vi "New Event Transport.vi"(10 "Event Priority (normal)":T1) -> (0 "error out":errorcluster, 2 "Tranport Event":refnum<user-event>, 3 "EventTransport Out":refnum<class "EventTransport.lvclass">)   [LabVIEW 2015, in "Mediator.lvlib" / "EventTransport.lvclass"]
doc: "<License>\nCopyright © 2017 Composed Systems, LLC | All rights reserved\nwww.composed.io\n\nAuthor: Ethan Stern <ethan.stern@composed.io>\n\nThis software is provided \"AS IS\" WITHOUT WARRANTIES, either express or implied, AND IS FOR EDUCATIONAL PURPOSES ONLY.\n</License>"
uses:
  EventTransport.lvclass
  <vilib>/event_ctls.llb/usereventprio.ctl
  EventTransport.lvclass/EventTransport.ctl
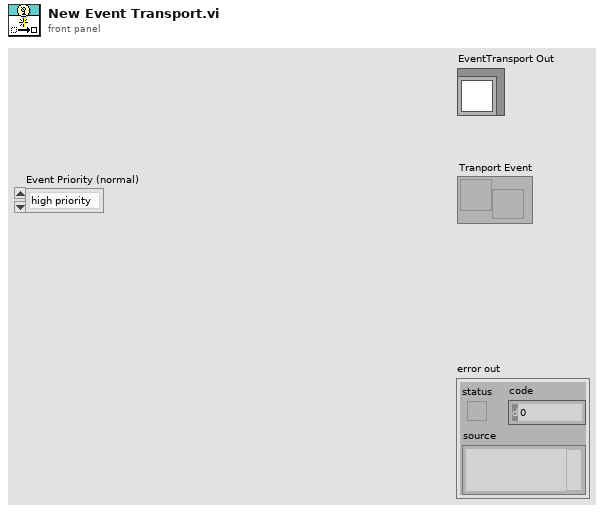
[diagram p1: front panel]
types:
  T1 = typedef "usereventprio.ctl" = enum32{"high priority", "normal priority"}
  T2 = cluster{"Data":variant, "Publication Time":timestamp}
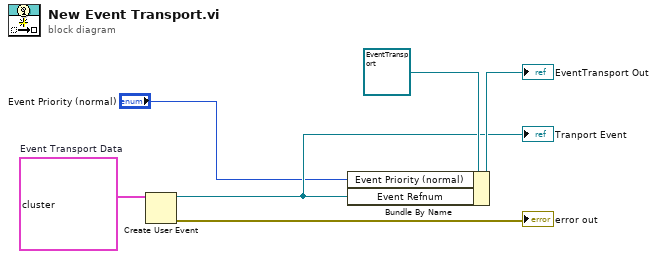
[diagram p0: block diagram]
diagram:
  w3 = T2 {"Data"=variant, "Publication Time"=timestamp(0 s since 1904-01-01)}  # Event Transport Data
  n1 = Create User Event(user event datatype=w3) -> (user event=w2:refnum<user-event>, error out=→"error out":errorcluster)  [unwired: 1 in]
  "Tranport Event" <- w2
  n2 = Bundle By Name(cluster=refnum<class "EventTransport.lvclass"> refnum ("ActorMessage in"), "Event Priority (normal)"="Event Priority (normal)", "Event Refnum"=w2) -> (→"EventTransport Out":refnum<class "EventTransport.lvclass">)
